vi "PassCmdEx.vi"(2 "超时毫秒(-1)":i32, 3 "cmd in":string, 4 "list ref":refnum<queue>) -> (0 "str out":string, 1 "cmd array out":string[](array[string]))   [LabVIEW 2012]
panel:
  out "new":bool
  in  "Msg":T1
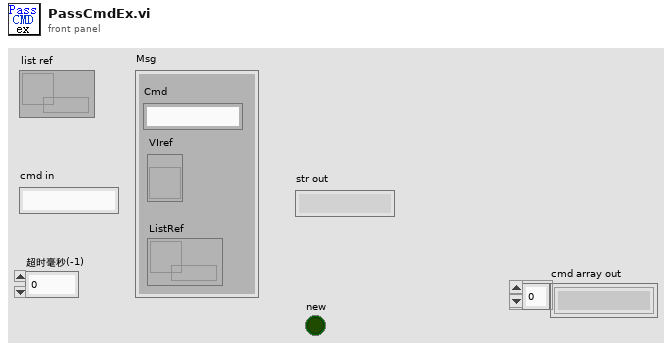
[diagram p1: front panel]
types:
  T1 = cluster{"Cmd":string, "VIref":refnum<vi>, "ListRef":refnum<queue>}
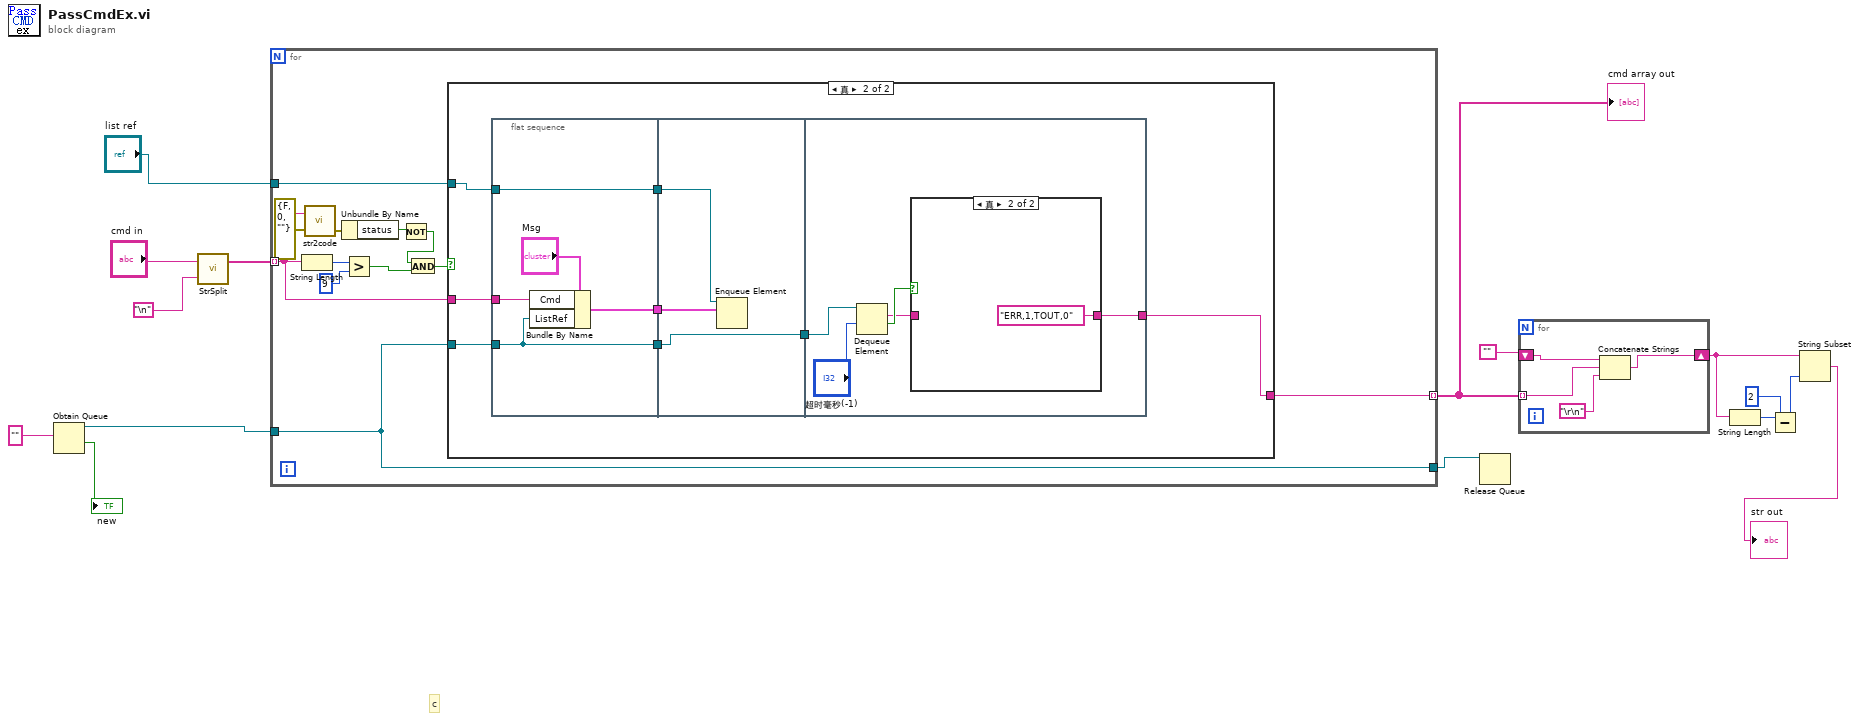
[diagram p0: block diagram]
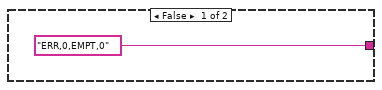
[diagram p2: hidden frame]
diagram:
  # "c"
  n1 = Obtain Queue(element data type="") -> (queue out=w11:refnum<queue>, created new?=→"new":bool)  [unwired: 4 in, 1 out]
  n2 = call "StrSplit.vi"("token"="\n", "str in"="cmd in") -> ("str out"=w14:string[])  [unwired: 1 out]
  n3 = for {
    tunnel: w14 -> [w22] mode=indexing
    tunnel: w11 -> [w23]
    tunnel: "list ref" -> [w27]
    tunnel: [w24] -> w7 mode=indexing
    tunnel: [w23] -> w9
    n4 = String Length(string=w22) -> (length=w26:i32)
    n5 = call "str2code.vi"("错误输入"=errorcluster {"status"=FALSE, "code"=0, "source"=""}, "input"=w22) -> ("error out"=w20:errorcluster)  [unwired: 1 out]
    n6 = Unbundle By Name(w20) -> ("status"=w19:bool)
    n7 = Greater?(x=w26, y=9) -> (0:w16:bool)
    n8 = Not(x=w19) -> (.not. x?=w17:bool)
    n9 = And(x=w17, y=w16) -> (x .and. y?=w18:bool)
    n10 = case shown="真" w18 {
      tunnel: w23 -> [_ w32]
      tunnel: w27 -> [_ w31]
      tunnel: ["ERR,0,EMPT,0" w29] -> w24
      tunnel: w22 -> [_ w30]
      frame False {
      }
      frame True {
        n11 = flat-sequence {
          tunnel: w31 -> [w41]
          tunnel: w32 -> [w38]
          tunnel: [w38] -> w36
          tunnel: [w41] -> w35
          tunnel: [w40] -> w34
          tunnel: w30 -> [w37]
          tunnel: [w44] -> w33
          tunnel: w36 -> [w44]
          tunnel: w35 -> [w43]
          tunnel: w34 -> [w42]
          tunnel: w33 -> [w49]
          tunnel: [w46] -> w29
          frame #0 {
            n12 = Bundle By Name(cluster="Msg", "Cmd"=w37, "ListRef"=w38) -> (w40:T1)
          }
          frame #1 {
            n13 = Enqueue Element(queue=w43, element=w42) -> ()  [unwired: 2 in, 3 out]
          }
          frame #2 {
            n14 = Dequeue Element(queue=w49, timeout in ms (-1)="超时毫秒(-1)") -> (element=w45:string, timed out?=w47:bool)  [unwired: 1 in, 2 out]
            n15 = case shown="真" w47 {
              tunnel: [w50 "ERR,1,TOUT,0"] -> w46
              tunnel: w45 -> [w50 _]
              frame False {
              }
              frame True {
              }
            }
          }
        }
      }
    }
  }
  "cmd array out" <- w7
  n16 = Release Queue(queue=w9) -> ()  [unwired: 2 in, 3 out]
  n17 = for {
    shift-right: [w52] -> w6
    shift-left: "" -> [w55]
    tunnel: w7 -> [w54] mode=indexing
    n18 = Concatenate Strings(w55, w54, "\r\n") -> (w52:string)
  }
  n19 = String Length(string=w6) -> (length=w5:i32)
  n20 = Subtract(x=w5, y=2) -> (x-y=w3:i32)
  n21 = String Subset(string=w6, length (rest)=w3) -> (substring=→"str out":string)  [unwired: 1 in]
